vi "log analysis_gps.vi"() -> ()   [LabVIEW 2018] (continued)
robot status\t98.646724\t124.090697\t7.903900\t-0.225779\t-0.330995\t22.927991\t0.293000\t0.000000\n\t\n15:11:22.4\tlog_raw\tgps_raw\t#DUALANTENNAHEADINGA,USB3,0,48.5,FINESTEERING,2107,281500.400,02008000,d426,15824;SOL_COMPUTED,L1_FLOAT,-1.000000000,46.407375336,-16.426940918,0.0,360.000000000,180.000000000,\"631T\",18,7,7,7,04,00,20,02*243e6382\n\tsystem status\tnormal 2 28.200000 0 0\trobot status\t98.785641\t124.138688\t7.903500\t-0.300068\t-0.288771\t22.729309\t0.300000\t0.001000\n\t\n15:11:22.9\tlog_raw\tgps_raw\t#DUALANTENNAHEADINGA,USB3,0,48.5,FINESTEERING,2107,281500.900,02008000,d426,15824;SOL_COMPUTED,L1_FLOAT,-1.000000000,46.192268372,-15.498413086,0.0,360.000000000,180.000000000,\"631T\",17,7,7,7,04,00,20,02*d63e23bb\n\tsystem status\tnormal 2 28.200000 0 0\trobot status\t98.919497\t124.181484\t7.902700\t-0.165116\t-0.303857\t22.510660\t0.296000\t-0.008000\n\t\n15:11:23.4\tlog_raw\tgps_raw\t#DUALANTENNAHEADINGA,USB3,0,48.5,FINESTEERING,2107,281501.400,02008000,d426,15824;SOL_COMPUTED,L1_FLOAT,-1.000000000,48.142848969,-21.188415527,0.0,360.000000000,180.000000000,\"631T\",17,7,7,7,04,00,20,02*7f9c1701\n\tsystem status\tnormal 2 28.200000 0 0\trobot status\t99.058497\t124.228185\t7.902400\t-0.026703\t-0.321474\t22.196441\t0.302000\t-0.008000\n\t\n15:11:23.9\tlog_raw\tgps_raw\t#DUALANTENNAHEADINGA,USB3,0,48.5,FINESTEERING,2107,281501.900,02008000,d426,15824;SOL_COMPUTED,L1_FLOAT,-1.000000000,48.243919373,-21.323577881,0.0,360.000000000,180.000000000,\"631T\",18,7,7,7,04,00,20,02*9b797559\n\tsystem status\tnormal 2 28.200000 0 0\trobot status\t99.198528\t124.274008\t7.901400\t0.031138\t-0.500462\t21.899605\t0.292000\t-0.018000\n\t\n15:11:24.4\tlog_raw\tgps_raw\t#DUALANTENNAHEADINGA,USB3,0,51.0,FINESTEERING,2107,281502.400,02000000,d426,15824;SOL_COMPUTED,L1_FLOAT,-1.000000000,54.417652130,-31.199645996,0.0,360.000000000,180.000000000,\"631T\",17,7,7,7,04,00,20,02*139cf8a7\n\tsystem status\tnormal 2 28.200000 0 0\trobot status\t99.336569\t124.322202\t7.900100\t-0.095211\t-0.669796\t21.458028\t0.235000\t-0.092000\n\t\n15:11:24.9\tlog_raw\tgps_raw\t\tsystem status\tnormal 2 28.100000 0 0\trobot status\t99.472138\t124.367009\t7.899200\t-0.169834\t-0.458120\t20.912602\t0.280000\t-0.035000\n\t\n15:11:25.4\tlog_raw\tgps_raw\t\tsystem status\tnormal 2 28.200000 0 0\trobot status\t99.609993\t124.411117\t7.898200\t-0.103974\t-0.294964\t20.251587\t0.290000\t-0.052000\n\t\n15:11:25.9\tlog_raw\tgps_raw\t\tsystem status\tnormal 2 28.100000 0 0\trobot status\t99.748652\t124.451922\t7.895200\t-0.029652\t-0.262619\t19.517331\t0.383000\t0.101000\n\t\n15:11:26.4\tlog_raw\tgps_raw\t\tsystem status\tnormal 2 28.100000 0 0\trobot status\t99.889419\t124.493856\t7.892100\t0.011105\t-0.261460\t18.582918\t0.286000\t-0.034000\n\t\n15:11:26.9\tlog_raw\tgps_raw\t#DUALANTENNAHEADINGA,USB3,0,51.0,FINESTEERING,2107,281504.900,02000000,d426,15824;SOL_COMPUTED,NARROW_FLOAT,-1.000000000,45.458030701,-24.170471191,0.0,349.614562988,180.000000000,\"631T\",18,7,7,7,04,00,20,03*3763f111\n\tsystem status\tnormal 2 28.000000 0 0\trobot status\t100.028200\t124.531303\t7.889700\t0.052509\t-0.445143\t17.486224\t0.246000\t-0.119000\n\t\n15:11:27.4\tlog_raw\tgps_raw\t\tsystem status\tnormal 2 28.000000 0 0\trobot status\t100.174107\t124.568549\t7.889400\t0.061035\t-0.832335\t16.254658\t0.300000\t-0.053000\n\t\n15:11:27.9\tlog_raw\tgps_raw\t\tsystem status\tnormal 2 28.000000 0 0\trobot status\t100.318986\t124.599317\t7.888100\t0.214199\t-1.050680\t15.191319\t0.290000\t-0.056000\n\t\n15:11:28.4\tlog_raw\tgps_raw\t#DUALANTENNAHEADINGA,USB3,0,47.0,FINESTEERING,2107,281506.400,02000000,d426,15824;SOL_COMPUTED,L1_FLOAT,-1.000000000,47.490772247,-15.120605469,0.0,360.000000000,180.000000000,\"631T\",20,7,7,7,04,00,20,02*6c842724\n\tsystem status\tnormal 2 28.000000 0 0\trobot status\t100.462357\t124.629809\t7.887200\t0.132799\t-1.007596\t14.087784\t0.295000\t-0.054000\n\t\n15:11:28.9\tlog_raw\tgps_raw\t#DUALANTENNAHEADINGA,USB3,0,47.0,FINESTEERING,2107,281506.900,02000000,d426,15824;SOL_COMPUTED,L1_FLOAT,-1.000000000,47.711154938,-15.635345459,0.0,360.000000000,180.000000000,\"631T\",18,7,7,7,04,00,20,02*a44c5d4d\n\tsystem status\tnormal 2 28.000000 0 0\trobot status\t100.606200\t124.656880\t7.884400\t-0.072719\t-0.959328\t13.073074\t0.251000\t-0.099000\n\t\n15:11:29.4\tlog_raw\tgps_raw\t#DUALANTENNAHEADINGA,USB3,0,47.5,FINESTEERING,2107,281507.400,02000000,d426,15824;SOL_COMPUTED,NARROW_FLOAT,-1.000000000,42.099899292,-18.667358398,0.0,341.481109619,180.000000000,\"631T\",17,7,7,7,04,00,20,03*b5db1bef\n\tsystem status\tnormal 2 28.000000 0 0\trobot status\t100.748865\t124.681433\t7.880500\t5.282500E-5\t-0.839396\t12.187824\t0.258000\t-0.078000\n\t\n15:11:29.9\tlog_raw\tgps_raw\t#INSPVAXA,USB3,0,47.5,FINESTEERING,2107,281507.950,02000000,471d,15824;INS_ALIGNMENT_COMPLETE,INS_RTKFIXED,37.37125380804,126.72197426812,7.8769,22.3000,-0.0203,0.2606,-0.0150,0.201245645,-0.677592145,78.627863448,0.4158,0.2828,0.5148,0.1162,0.0939,0.0753,0.2087,0.2003,5.2095,0f000001,0*4e226b57\n\tsystem status\tnormal 2 28.000000 0 0\trobot status\t100.905195\t124.702970\t7.876900\t0.201246\t-0.677592\t11.372137\t0.348000\t0.066000\n\t\n15:11:30.4\tlog_raw\tgps_raw\t\tsystem status\tnormal 2 28.000000 0 0\trobot status\t101.036080\t124.720598\t7.875000\t0.298084\t-0.652481\t10.723363\t0.297000\t-0.011000\n\t\n15:11:30.9\tlog_raw\tgps_raw\t#DUALANTENNAHEADINGA,USB3,0,49.0,FINESTEERING,2107,281508.900,02000000,d426,15824;SOL_COMPUTED,L1_FLOAT,-1.000000000,44.870548248,-15.658569336,0.0,360.000000000,180.000000000,\"631T\",16,7,7,7,04,00,20,02*b0c8f4ea\n\tsystem status\tnormal 2 28.100000 0 0\trobot status\t101.181077\t124.738550\t7.872400\t0.183203\t-0.630905\t10.014511\t0.311000\t0.003000\n\t\n15:11:31.4\tlog_raw\tgps_raw\t#DUALANTENNAHEADINGA,USB3,0,48.0,FINESTEERING,2107,281509.400,02000000,d426,15824;SOL_COMPUTED,NARROW_FLOAT,-1.000000000,43.414321899,-11.001037598,0.0,331.000732422,180.000000000,\"631T\",16,7,7,7,04,00,20,03*47deaf74\n\tsystem status\tnormal 2 28.100000 0 0\trobot status\t101.323239\t124.757427\t7.870200\t0.032270\t-0.532308\t9.546934\t0.287000\t-0.036000\n\t\n15:11:31.9\tlog_raw\tgps_raw\t#INSPVAXA,USB3,0,48.0,FINESTEERING,2107,281509.950,02000000,471d,15824;INS_ALIGNMENT_COMPLETE,INS_RTKFIXED,37.37125445097,126.72198074425,7.8673,22.3000,-0.0085,0.2660,-0.0026,-0.121772207,-0.607137029,81.065804036,0.4154,0.2822,0.5141,0.1167,0.0945,0.0753,0.2051,0.1982,5.2122,0f000001,0*3f1eba48\n\tsystem status\tnormal 2 28.100000 0 0\trobot status\t101.478840\t124.774319\t7.867300\t-0.121772\t-0.607137\t8.934196\t0.256000\t-0.074000\n\t\n15:11:32.4\tlog_raw\tgps_raw\t\tsystem status\tnormal 2 28.200000 0 0\trobot status\t101.608572\t124.787896\t7.865000\t0.007019\t-0.726552\t8.514396\t0.304000\t-0.013000\n\t\n15:11:32.9\tlog_raw\tgps_raw\t#INSPVAXA,USB3,0,49.0,FINESTEERING,2107,281510.950,02000000,471d,15824;INS_ALIGNMENT_COMPLETE,INS_RTKFIXED,37.37125469386,126.72198394017,7.8637,22.3000,-0.0196,0.2391,0.0072,0.076200497,-0.660108168,81.872681824,0.4156,0.2817,0.5136,0.1168,0.0948,0.0753,0.2032,0.1971,5.2137,0f000001,0*0481949b\n\tsystem status\tnormal 2 28.200000 0 0\trobot status\t101.761929\t124.801272\t7.863700\t0.076200\t-0.660108\t8.127318\t0.235000\t-0.092000\n\t\n15:11:33.4\tlog_raw\tgps_raw\t#DUALANTENNAHEADINGA,USB3,0,46.5,FINESTEERING,2107,281511.400,02000000,d426,15824;SOL_COMPUTED,L1_FLOAT,-1.000000000,48.665706635,-11.851898193,0.0,360.000000000,180.000000000,\"631T\",23,7,7,7,04,00,20,02*002e390f\n\tsystem status\tnormal 2 28.200000 0 0\trobot status\t101.889941\t124.812552\t7.861000\t0.084258\t-0.827369\t7.753561\t0.346000\t0.053000\n\t\n15:11:33.9\tlog_raw\tgps_raw\t#DUALANTENNAHEADINGA,USB3,0,46.5,FINESTEERING,2107,281511.900,02000000,d426,15824;SOL_COMPUTED,L1_FLOAT,-1.000000000,49.675540924,-13.921539307,0.0,360.000000000,180.000000000,\"631T\",22,7,7,7,04,00,20,02*d8f1bbd6\n\tsystem status\tnormal 2 28.200000 0 0\trobot status\t102.034901\t124.823355\t7.857600\t0.091248\t-1.206859\t7.443421\t0.347000\t0.065000\n\t\n15:11:34.4\tlog_raw\tgps_raw\t\tsystem status\tnormal 2 28.200000 0 0\trobot status\t102.180454\t124.835621\t7.854200\t0.123162\t-1.430289\t7.169938\t0.298000\t-0.010000\n\t\n15:11:34.9\tlog_raw\tgps_raw\t\tsystem status\tnormal 2 28.200000 0 0\trobot status\t102.318034\t124.846412\t7.851300\t0.027853\t-1.487298\t6.927742\t0.312000\t-0.001000\n\t\n15:11:35.4\tlog_raw\tgps_raw\t\tsystem status\tnormal 2 28.200000 0 0\trobot status\t102.466690\t124.857181\t7.847700\t0.249609\t-1.679451\t6.774904\t0.306000\t-0.003000\n\t\n15:11:35.9\tlog_raw\tgps_raw\t#DUALANTENNAHEADINGA,USB3,0,49.5,FINESTEERING,2107,281513.900,02000000,d426,15824;SOL_COMPUTED,NARROW_FLOAT,-1.000000000,44.284626007,-19.218811035,0.0,360.000000000,180.000000000,\"631T\",20,7,7,7,04,00,20,02*521f05df\n\tsystem status\tnormal 2 28.200000 0 0\trobot status\t102.608975\t124.865714\t7.841900\t0.369371\t-1.895271\t6.487621\t0.281000\t-0.030000\n\t\n15:11:36.4\tlog_raw\tgps_raw\t#INSPVAXA,USB3,0,49.5,FINESTEERING,2107,281514.450,02000000,471d,15824;INS_ALIGNMENT_COMPLETE,INS_RTKFIXED,37.37125536287,126.72199528915,7.8355,22.3000,-0.0378,0.2111,0.0002,0.439353966,-1.869293948,83.706823159,0.4159,0.2810,0.5124,0.1164,0.0945,0.0753,0.1954,0.1923,5.2170,0f000001,0*665bd911\n\tsystem status\tnormal 2 28.200000 0 0\trobot status\t102.767204\t124.875510\t7.835500\t0.439354\t-1.869294\t6.293177\t0.346000\t0.076000\n\t\n15:11:36.9\tlog_raw\tgps_raw\t\tsystem status\tnormal 2 28.200000 0 0\trobot status\t102.889412\t124.880327\t7.832000\t0.623351\t-1.525820\t6.078909\t0.311000\t-0.001000\n\t\n15:11:37.4\tlog_raw\tgps_raw\t#DUALANTENNAHEADINGA,USB3,0,49.0,FINESTEERING,2107,281515.400,02000000,d426,15824;SOL_COMPUTED,L1_FLOAT,-1.000000000,38.143417358,-18.359069824,0.0,274.915802002,180.000000000,\"631T\",19,9,9,9,04,00,20,22*781bfffa\n\tsystem status\tnormal 2 28.200000 0 0\trobot status\t103.038346\t124.886833\t7.827900\t0.687382\t-1.870260\t5.833892\t0.299000\t-0.009000\n\t\n15:11:37.9\tlog_raw\tgps_raw\t#INSPVAXA,USB3,0,49.0,FINESTEERING,2107,281515.950,02000000,471d,15824;INS_ALIGNMENT_COMPLETE,INS_RTKFIXED,37.37125550223,126.72200026219,7.8204,22.3000,-0.0297,0.2447,-0.0075,0.993050035,-2.146972664,84.455014366,0.4154,0.2808,0.5121,0.1158,0.0940,0.0753,0.1936,0.1911,5.2166,0f000001,0*f4a4a55a\n\tsystem status\tnormal 2 28.200000 0 0\trobot status\t103.207707\t124.890971\t7.820400\t0.993050\t-2.146973\t5.544986\t0.330000\t0.040000\n\t\n15:11:38.4\tlog_raw\tgps_raw\t\tsystem status\tnormal 2 28.200000 0 0\trobot status\t103.325362\t124.896784\t7.815000\t0.884537\t-1.973530\t5.489952\t0.303000\t-0.002000\n\t\n15:11:38.9\tlog_raw\tgps_raw\t#INSPVAXA,USB3,0,49.5,FINESTEERING,2107,281516.950,02000000,471d,15824;INS_ALIGNMENT_COMPLETE,INS_RTKFIXED,37.37125561676,126.72200346260,7.8093,22.3000,-0.0298,0.2388,-0.0036,0.877000312,-2.356206716,84.738207188,0.4150,0.2807,0.5119,0.1151,0.0935,0.0753,0.1918,0.1900,5.2169,0f000001,0*302168dd\n\tsystem status\tnormal 2 28.200000 0 0\trobot status\t103.491194\t124.903679\t7.809300\t0.877000\t-2.356207\t5.261793\t0.283000\t-0.020000\n\t\n15:11:39.4\tlog_raw\tgps_raw\t\tsystem status\tnormal 2 28.200000 0 0\trobot status\t103.620894\t124.907401\t7.804000\t1.139173\t-2.452817\t5.195560\t0.315000\t0.002000\n\t\n15:11:39.9\tlog_raw\tgps_raw\t#INSPVAXA,USB3,0,49.0,FINESTEERING,2107,281517.950,02000000,471d,15824;INS_ALIGNMENT_COMPLETE,INS_RTKFIXED,37.37125568444,126.72200682151,7.7945,22.3000,-0.0192,0.2217,-0.0192,1.425946451,-2.539207007,85.090836671,0.4150,0.2807,0.5120,0.1146,0.0931,0.0754,0.1902,0.1890,5.2177,0f000001,0*9a7264e1\n\tsystem status\tnormal 2 28.200000 0 0\trobot status\t103.788721\t124.911187\t7.794500\t1.425946\t-2.539207\t4.909163\t0.292000\t-0.003000\n\t\n15:11:40.4\tlog_raw\tgps_raw\t#DUALANTENNAHEADINGA,USB3,0,47.0,FINESTEERING,2107,281518.400,02000000,d426,15824;SOL_COMPUTED,L1_FLOAT,-1.000000000,42.740367889,-32.075164795,0.0,319.860687256,180.000000000,\"631T\",19,9,9,9,04,00,20,22*d53a90ac\n\tsystem status\tnormal 2 28.200000 0 0\trobot status\t103.913646\t124.913656\t7.788400\t1.548086\t-2.511237\t4.765725\t0.294000\t-0.015000\n\t\n15:11:40.9\tlog_raw\tgps_raw\t#INSPVAXA,USB3,0,47.0,FINESTEERING,2107,281518.950,02000000,471d,15824;INS_ALIGNMENT_COMPLETE,INS_RTKFIXED,37.37125573981,126.72201005340,7.7819,22.3000,-0.0255,0.2627,-0.0105,1.331964681,-2.358060852,85.490717042,0.4145,0.2807,0.5123,0.1139,0.0926,0.0754,0.1888,0.1882,5.2187,0f000001,0*a7b8d42f\n\tsystem status\tnormal 2 28.200000 0 0\trobot status\t104.074997\t124.917328\t7.781900\t1.331965\t-2.358061\t4.509283\t0.295000\t-0.010000\n\t\n15:11:41.4\tlog_raw\tgps_raw\t\tsystem status\tnormal 2 28.200000 0 0\trobot status\t104.206873\t124.921189\t7.776100\t1.272173\t-2.469468\t4.361029\t0.303000\t-0.005000\n\t\n15:11:41.9\tlog_raw\tgps_raw\t#DUALANTENNAHEADINGA,USB3,0,48.5,FINESTEERING,2107,281519.900,02000000,d426,15824;SOL_COMPUTED,L1_FLOAT,-1.000000000,50.327861786,-37.477569580,0.0,318.157135010,180.000000000,\"631T\",19,6,6,6,04,00,20,02*633b419f\n\tsystem status\tnormal 2 28.200000 0 0\trobot status\t104.351513\t124.926330\t7.769800\t0.918221\t-2.120112\t4.233972\t0.281000\t-0.028000\n\t\n15:11:42.4\tlog_raw\tgps_raw\t#INSPVAXA,USB3,0,50.5,FINESTEERING,2107,281520.450,02000000,471d,15824;INS_ALIGNMENT_COMPLETE,INS_RTKFIXED,37.37125585823,126.72201493380,7.7618,22.3000,-0.0241,0.3156,-0.0229,0.726950226,-1.736335122,85.946194280,0.4135,0.2799,0.5121,0.1130,0.0919,0.0756,0.1864,0.1868,5.2210,0f000001,0*82c9f176\n\tsystem status\tnormal 2 28.200000 0 0\trobot status\t104.507294\t124.930466\t7.761800\t0.726950\t-1.736335\t4.053806\t0.309000\t-0.011000\n\t\n15:11:42.9\tlog_raw\tgps_raw\t#INSPVAXA,USB3,0,50.5,FINESTEERING,2107,281520.950,02000000,471d,15824;INS_ALIGNMENT_COMPLETE,INS_RTKFIXED,37.37125587974,126.72201671987,7.7507,22.3000,-0.0399,0.2427,-0.0046,0.656221205,-1.866737279,86.202077970,0.4135,0.2799,0.5121,0.1130,0.0919,0.0756,0.1864,0.1868,5.2210,0f000001,0*df1ef1f5\n\tsystem status\tnormal 2 28.200000 0 0\trobot status\t104.665502\t124.932851\t7.750700\t0.656221\t-1.866737\t3.797922\t0.277000\t-0.018000\n\t\n15:11:43.4\tlog_raw\tgps_raw\t\tsystem status\tnormal 2 28.200000 0 0\trobot status\t104.773354\t124.932494\t7.745800\t0.650732\t-1.574531\t3.665864\t0.288000\t0.009000\n\t\n15:11:43.9\tlog_raw\tgps_raw\t#INSPVAXA,USB3,0,46.5,FINESTEERING,2107,281521.950,02000000,471d,15824;INS_ALIGNMENT_COMPLETE,INS_RTKFIXED,37.37125587376,126.72201976127,7.7406,22.3000,-0.0074,0.2755,0.0027,0.545815584,-0.620038116,86.574318389,0.4139,0.2794,0.5123,0.1122,0.0918,0.0756,0.1854,0.1863,5.2222,0f000001,0*d388b8b0\n\tsystem status\tnormal 2 28.200000 0 0\trobot status\t104.934904\t124.932184\t7.740600\t0.545816\t-0.620038\t3.425682\t0.297000\t-0.002000\n\t\n15:11:44.4\tlog_raw\tgps_raw\t#INSPVAXA,USB3,0,50.0,FINESTEERING,2107,281522.450,02000000,471d,15824;INS_ALIGNMENT_COMPLETE,INS_RTKFIXED,37.37125594460,126.72202128419,7.7372,22.3000,-0.0117,0.2731,-0.0129,-0.654259534,-0.666330623,86.875849096,0.4136,0.2787,0.5123,0.1124,0.0922,0.0756,0.1845,0.1859,5.2224,0f000001,0*d87bbb5d\n\tsystem status\tnormal 2 28.200000 0 0\trobot status\t105.069802\t124.940044\t7.737200\t-0.654260\t-0.666331\t3.124151\t0.300000\t0.002000\n\t\n15:11:44.9\tlog_raw\tgps_raw\t#INSPVAXA,USB3,0,50.0,FINESTEERING,2107,281522.950,02000000,471d,15824;INS_ALIGNMENT_COMPLETE,INS_RTKFIXED,37.37125596414,126.72202295836,7.7342,22.3000,-0.0333,0.2828,-0.0046,-1.065587948,-0.382081597,87.029767697,0.4136,0.2787,0.5123,0.1124,0.0922,0.0756,0.1845,0.1859,5.2224,0f000001,0*2edab05f\n\tsystem status\tnormal 2 28.200000 0 0\trobot status\t105.218097\t124.942211\t7.734200\t-1.065588\t-0.382082\t2.970232\t0.302000\t-0.002000\n\t\n15:11:45.4\tlog_raw\tgps_raw\t#INSPVAXA,USB3,0,50.0,FINESTEERING,2107,281523.450,02000000,471d,15824;INS_ALIGNMENT_COMPLETE,INS_RTKFIXED,37.37125596415,126.72202454079,7.7319,22.3000,-0.0484,0.2411,-0.0123,-1.089747503,0.421440588,87.147048457,0.4141,0.2781,0.5123,0.1124,0.0923,0.0755,0.1837,0.1856,5.2192,0f000001,0*53e95b2b\n\tsystem status\tnormal 2 28.200000 0 0\trobot status\t105.358266\t124.942210\t7.731900\t-1.089748\t0.421441\t2.852952\t0.294000\t0.001000\n\t\n15:11:45.9\tlog_raw\tgps_raw\t#INSPVAXA,USB3,0,50.0,FINESTEERING,2107,281523.950,02000000,471d,15824;INS_ALIGNMENT_COMPLETE,INS_RTKFIXED,37.37125592914,126.72202612283,7.7345,22.3000,-0.0454,0.2984,-0.0075,-0.788968159,0.571056615,87.325442989,0.4141,0.2781,0.5123,0.1124,0.0923,0.0755,0.1837,0.1856,5.2192,0f000001,0*39ccc3b7\n\tsystem status\tnormal 2 28.200000 0 0\trobot status\t105.498400\t124.938323\t7.734500\t-0.788968\t0.571057\t2.674557\t0.312000\t-0.009000\n\t\n15:11:46.4\tlog_raw\tgps_raw\t#INSPVAXA,USB3,0,50.0,FINESTEERING,2107,281524.450,02000000,471d,15824;INS_ALIGNMENT_COMPLETE,INS_RTKFIXED,37.37125593181,126.72202769254,7.7370,22.3000,-0.0382,0.2867,-0.0035,-1.197739356,0.920892759,87.655051313,0.4147,0.2775,0.5122,0.1123,0.0915,0.0754,0.1830,0.1854,5.2111,0f000001,0*f9d72c69\n\tsystem status\tnormal 2 28.200000 0 0\trobot status\t105.637443\t124.938618\t7.737000\t-1.197739\t0.920893\t2.344949\t0.309000\t-0.005000\n\t\n15:11:46.9\tlog_raw\tgps_raw\t#INSPVAXA,USB3,0,50.0,FINESTEERING,2107,281524.950,02000000,471d,15824;INS_ALIGNMENT_COMPLETE,INS_RTKFIXED,37.37125591109,126.72202930356,7.7399,22.3000,-0.0391,0.2791,0.0008,-1.548464832,1.177525409,87.896240869,0.4147,0.2775,0.5122,0.1123,0.0915,0.0754,0.1830,0.1854,5.2111,0f000001,0*83d571d9\n\tsystem status\tnormal 2 28.200000 0 0\trobot status\t105.780144\t124.936316\t7.739900\t-1.548465\t1.177525\t2.103759\t0.307000\t-0.003000\n\t\n15:11:47.4\tlog_raw\tgps_raw\t\tsystem status\tnormal 2 28.200000 0 0\trobot status\t105.910401\t124.935971\t7.743500\t-1.684978\t1.371222\t1.943675\t0.296000\t0.003000\n\t\n15:11:47.9\tlog_raw\tgps_raw\t\tsystem status\tnormal 2 28.200000 0 0\trobot status\t106.056063\t124.933146\t7.747400\t-1.614315\t1.306008\t1.765428\t0.294000\t0.000000\n\t\n15:11:48.4\tlog_raw\tgps_raw\t#INSPVAXA,USB3,0,48.5,FINESTEERING,2107,281526.450,02000000,471d,15824;INS_ALIGNMENT_COMPLETE,INS_RTKFIXED,37.37125584524,126.72203425117,7.7504,22.3000,-0.0601,0.2713,0.0036,-1.381885120,0.929156206,88.315257538,0.4157,0.2770,0.5121,0.1113,0.0909,0.0752,0.1819,0.1851,5.1872,0f000001,0*291f5036\n\tsystem status\tnormal 2 28.200000 0 0\trobot status\t106.218395\t124.929002\t7.750400\t-1.381885\t0.929156\t1.684742\t0.293000\t-0.004000\n\t\n15:11:48.9\tlog_raw\tgps_raw\t#INSPVAXA,USB3,0,48.5,FINESTEERING,2107,281526.950,02000000,471d,15824;INS_ALIGNMENT_COMPLETE,INS_RTKFIXED,37.37125579589,126.72203592362,7.7537,22.3000,-0.0480,0.2913,0.0058,-1.173614643,0.491373435,88.468098550,0.4157,0.2770,0.5121,0.1113,0.0909,0.0752,0.1819,0.1851,5.1872,0f000001,0*d2925fbc\n\tsystem status\tnormal 2 28.200000 0 0\trobot status\t106.366538\t124.923523\t7.753700\t-1.173615\t0.491373\t1.531901\t0.306000\t0.008000\n\t\n15:11:49.4\tlog_raw\tgps_raw\t\tsystem status\tnormal 2 28.200000 0 0\trobot status\t106.498057\t124.921350\t7.758600\t-1.119985\t0.342214\t1.463884\t0.297000\t0.006000\n\t\n15:11:49.9\tlog_raw\tgps_raw\t#INSPVAXA,USB3,0,48.0,FINESTEERING,2107,281527.950,02000000,471d,15824;INS_ALIGNMENT_COMPLETE,INS_RTKFIXED,37.37125572987,126.72203920387,7.7658,22.3000,-0.0524,0.2827,0.0097,-1.037615200,0.271270878,88.658127603,0.4153,0.2771,0.5121,0.1104,0.0905,0.0752,0.1816,0.1850,5.1752,0f000001,0*cc65e324\n\tsystem status\tnormal 2 28.200000 0 0\trobot status\t106.657097\t124.916193\t7.765800\t-1.037615\t0.271271\t1.341872\t0.302000\t0.006000\n\t\n15:11:50.4\tlog_raw\tgps_raw\t#INSPVAXA,USB3,0,50.0,FINESTEERING,2107,281528.450,02000000,471d,15824;INS_ALIGNMENT_COMPLETE,INS_RTKFIXED,37.37125569644,126.72204084208,7.7707,22.3000,-0.0559,0.2951,0.0043,-0.934405455,0.587306829,88.715451510,0.4138,0.2768,0.5118,0.1101,0.0902,0.0751,0.1812,0.1850,5.1681,0f000001,0*38aa8fdd\n\tsystem status\tnormal 2 28.200000 0 0\trobot status\t106.802207\t124.912480\t7.770700\t-0.934405\t0.587307\t1.284548\t0.301000\t0.002000\n\t\n15:11:50.9\tlog_raw\tgps_raw\t#INSPVAXA,USB3,0,50.0,FINESTEERING,2107,281528.950,02000000,471d,15824;INS_ALIGNMENT_COMPLETE,INS_RTKFIXED,37.37125565087,126.72204247728,7.7739,22.3000,-0.0479,0.2916,0.0001,-0.888338031,0.781445457,88.804413207,0.4138,0.2768,0.5118,0.1101,0.0902,0.0751,0.1812,0.1850,5.1681,0f000001,0*a995e794\n\tsystem status\tnormal 2 28.200000 0 0\trobot status\t106.947051\t124.907421\t7.773900\t-0.888338\t0.781445\t1.195587\t0.298000\t0.004000\n\t\n15:11:51.4\tlog_raw\tgps_raw\t#INSPVAXA,USB3,0,45.5,FINESTEERING,2107,281529.450,02000000,471d,15824;INS_ALIGNMENT_COMPLETE,INS_RTKFIXED,37.37125561815,126.72204405961,7.7805,22.3000,-0.0427,0.2707,0.0059,-0.985512427,0.998310951,88.869085357,0.4125,0.2769,0.5116,0.1099,0.0902,0.0751,0.1810,0.1850,5.1659,0f000001,0*0269fb35\n\tsystem status\tnormal 2 28.200000 0 0\trobot status\t107.087211\t124.903788\t7.780500\t-0.985512\t0.998311\t1.130915\t0.294000\t-0.009000\n\t\n15:11:51.9\tlog_raw\tgps_raw\t#INSPVAXA,USB3,0,45.5,FINESTEERING,2107,281529.950,02000000,471d,15824;INS_ALIGNMENT_COMPLETE,INS_RTKFIXED,37.37125556208,126.72204568853,7.7886,22.3000,-0.0448,0.2875,0.0039,-0.937316119,0.971606302,88.876668498,0.4125,0.2769,0.5116,0.1099,0.0902,0.0751,0.1810,0.1850,5.1659,0f000001,0*914c1aec\n\tsystem status\tnormal 2 28.200000 0 0\trobot status\t107.231498\t124.897563\t7.788600\t-0.937316\t0.971606\t1.123332\t0.298000\t-0.003000\n\t\n15:11:52.4\tlog_raw\tgps_raw\t#INSPVAXA,USB3,0,49.0,FINESTEERING,2107,281530.450,02000000,471d,15824;INS_ALIGNMENT_COMPLETE,INS_RTKFIXED,37.37125551286,126.72204733678,7.7958,22.3000,-0.0391,0.2940,0.0024,-0.847859787,0.758698314,88.842002918,0.4116,0.2768,0.5112,0.1098,0.0901,0.0751,0.1808,0.1849,5.1659,0f000001,0*a7731e83\n\tsystem status\tnormal 2 28.200000 0 0\trobot status\t107.377497\t124.892099\t7.795800\t-0.847860\t0.758698\t1.157997\t0.300000\t0.001000\n\t\n15:11:52.9\tlog_raw\tgps_raw\t#INSPVAXA,USB3,0,49.0,FINESTEERING,2107,281530.950,02000000,471d,15824;INS_ALIGNMENT_COMPLETE,INS_RTKFIXED,37.37125545025,126.72204900061,7.8022,22.3000,-0.0360,0.2787,-0.0016,-0.812645512,0.794768831,88.914177046,0.4116,0.2768,0.5112,0.1098,0.0901,0.0751,0.1808,0.1849,5.1659,0f000001,0*55377a3b\n\tsystem status\tnormal 2 28.200000 0 0\trobot status\t107.524877\t124.885148\t7.802200\t-0.812646\t0.794769\t1.085823\t0.296000\t0.003000\n\t\n15:11:53.4\tlog_raw\tgps_raw\t#INSPVAXA,USB3,0,48.5,FINESTEERING,2107,281531.450,02000000,471d,15824;INS_ALIGNMENT_COMPLETE,INS_RTKFIXED,37.37125540137,126.72205063289,7.8075,22.3000,-0.0425,0.2797,0.0032,-0.889554517,0.869596367,88.992176965,0.4129,0.2847,0.5220,0.1101,0.0915,0.0760,0.1808,0.1849,5.1672,0f000001,0*7c4913e5\n\tsystem status\tnormal 2 28.200000 0 0\trobot status\t107.669461\t124.879721\t7.807500\t-0.889555\t0.869596\t1.007823\t0.302000\t0.002000\n\t\n15:11:53.9\tlog_raw\tgps_raw\t#INSPVAXA,USB3,0,48.5,FINESTEERING,2107,281531.950,02000000,471d,15824;INS_ALIGNMENT_COMPLETE,INS_RTKFIXED,37.37125534314,126.72205229379,7.8137,22.3000,-0.0465,0.3065,0.0071,-1.008380878,0.751327706,89.074001876,0.4129,0.2847,0.5220,0.1101,0.0915,0.0760,0.1808,0.1849,5.1672,0f000001,0*42202879\n\tsystem status\tnormal 2 28.200000 0 0\trobot status\t107.816581\t124.873257\t7.813700\t-1.008381\t0.751328\t0.925998\t0.302000\t0.002000\n\t\n15:11:54.4\tlog_raw\tgps_raw\t#INSPVAXA,USB3,0,47.5,FINESTEERING,2107,281532.450,02000000,471d,15824;INS_ALIGNMENT_COMPLETE,INS_RTKFIXED,37.37125529086,126.72205393210,7.8208,22.3000,-0.0380,0.2964,0.0024,-1.066354382,0.654899534,89.120116128,0.4138,0.2906,0.5321,0.1104,0.0921,0.0766,0.1807,0.1849,5.1689,0f000001,0*be946886\n\tsystem status\tnormal 2 28.200000 0 0\trobot status\t107.961700\t124.867452\t7.820800\t-1.066354\t0.654900\t0.879884\t0.299000\t0.003000\n\t\n15:11:54.9\tlog_raw\tgps_raw\t#INSPVAXA,USB3,0,47.5,FINESTEERING,2107,281532.950,02000000,471d,15824;INS_ALIGNMENT_COMPLETE,INS_RTKFIXED,37.37125523061,126.72205555403,7.8287,22.3000,-0.0378,0.2817,0.0049,-1.169453281,0.642583735,89.146408526,0.4138,0.2906,0.5321,0.1104,0.0921,0.0766,0.1807,0.1849,5.1689,0f000001,0*6f8607ae\n\tsystem status\tnormal 2 28.200000 0 0\trobot status\t108.105368\t124.860764\t7.828700\t-1.169453\t0.642584\t0.853591\t0.295000\t0.002000\n\t\n15:11:55.4\tlog_raw\tgps_raw\t#INSPVAXA,USB3,0,48.5,FINESTEERING,2107,281533.450,02000000,471d,15824;INS_ALIGNMENT_COMPLETE,INS_RTKFIXED,37.37125517665,126.72205724840,7.8341,22.3000,-0.0370,0.2921,0.0139,-1.096637131,0.532202635,89.160335545,0.4113,0.2846,0.5267,0.1101,0.0906,0.0761,0.1804,0.1849,5.1704,0f000001,0*30c8b167\n\tsystem status\tnormal 2 28.200000 0 0\trobot status\t108.255452\t124.854773\t7.834100\t-1.096637\t0.532203\t0.839664\t0.304000\t0.000000\n\t\n15:11:55.9\tlog_raw\tgps_raw\t#INSPVAXA,USB3,0,48.5,FINESTEERING,2107,281533.950,02000000,471d,15824;INS_ALIGNMENT_COMPLETE,INS_RTKFIXED,37.37125511841,126.72205890911,7.8393,22.3000,-0.0280,0.2944,0.0195,-1.130148525,0.576717755,89.139209909,0.4113,0.2846,0.5267,0.1101,0.0906,0.0761,0.1804,0.1849,5.1704,0f000001,0*9cf16a0c\n\tsystem status\tnormal 2 28.200000 0 0\trobot status\t108.402555\t124.848307\t7.839300\t-1.130149\t0.576718\t0.860790\t0.304000\t-0.003000\n\t\n15:11:56.4\tlog_raw\tgps_raw\t#INSPVAXA,USB3,0,49.0,FINESTEERING,2107,281534.450,02000000,471d,15824;INS_ALIGNMENT_COMPLETE,INS_RTKFIXED,37.37125507853,126.72206052520,7.8451,22.3000,-0.0278,0.2839,0.0233,-1.120245446,0.696634414,89.152346595,0.4098,0.2808,0.5226,0.1101,0.0900,0.0757,0.1802,0.1849,5.1715,0f000001,0*4ae7b9de\n\tsystem status\tnormal 2 28.200000 0 0\trobot status\t108.545706\t124.843880\t7.845100\t-1.120245\t0.696634\t0.847653\t0.278000\t0.038000\n\t\n15:11:56.9\tlog_raw\tgps_raw\t\tsystem status\tnormal 2 28.200000 0 0\trobot status\t108.675907\t124.839047\t7.850800\t-1.049400\t0.685732\t0.841710\t0.256000\t0.060000\n\t\n15:11:57.4\tlog_raw\tgps_raw\t#INSPVAXA,USB3,0,48.5,FINESTEERING,2107,281535.450,02000000,471d,15824;INS_ALIGNMENT_COMPLETE,INS_RTKFIXED,37.37125500223,126.72206378998,7.8595,22.3000,-0.0263,0.2848,0.0309,-1.021616386,0.668311678,89.031237589,0.4086,0.2786,0.5193,0.1098,0.0898,0.0755,0.1801,0.1849,5.1718,0f000001,0*96cd35cb\n\tsystem status\tnormal 2 28.200000 0 0\trobot status\t108.834895\t124.835408\t7.859500\t-1.021616\t0.668312\t0.968762\t0.295000\t0.014000\n\t\n15:11:57.9\tlog_raw\tgps_raw\t#INSPVAXA,USB3,0,48.5,FINESTEERING,2107,281535.950,02000000,471d,15824;INS_ALIGNMENT_COMPLETE,INS_RTKFIXED,37.37125496736,126.72206538562,7.8673,22.3000,-0.0208,0.2826,0.0283,-0.984984816,0.649258027,88.926389870,0.4086,0.2786,0.5193,0.1098,0.0898,0.0755,0.1801,0.1849,5.1718,0f000001,0*d651761b\n\tsystem status\tnormal 2 28.200000 0 0\trobot status\t108.976234\t124.831536\t7.867300\t-0.984985\t0.649258\t1.073610\t0.295000\t0.021000\n\t\n15:11:58.4\tlog_raw\tgps_raw\t#INSPVAXA,USB3,0,43.0,FINESTEERING,2107,281536.450,02000000,471d,15824;INS_ALIGNMENT_COMPLETE,INS_RTKFIXED,37.37125494902,126.72206698066,7.8731,22.3000,-0.0263,0.2809,0.0211,-1.040366850,0.673880913,88.812825832,0.4080,0.2774,0.5168,0.1098,0.0898,0.0754,0.1801,0.1849,5.1719,0f000001,0*bc17f841\n\tsystem status\tnormal 2 28.200000 0 0\trobot status\t109.117520\t124.829498\t7.873100\t-1.040367\t0.673881\t1.187174\t0.354000\t-0.072000\n\t\n15:11:58.9\tlog_raw\tgps_raw\t#INSPVAXA,USB3,0,43.0,FINESTEERING,2107,281536.950,02000000,471d,15824;INS_ALIGNMENT_COMPLETE,INS_RTKFIXED,37.37125492336,126.72206864315,7.8782,22.3000,-0.0243,0.2721,0.0164,-1.054954219,0.518295221,88.745495992,0.4080,0.2774,0.5168,0.1098,0.0898,0.0754,0.1801,0.1849,5.1719,0f000001,0*93a4c9d5\n\tsystem status\tnormal 2 28.200000 0 0\trobot status\t109.264781\t124.826649\t7.878200\t-1.054954\t0.518295\t1.254504\t0.285000\t0.018000\n\t\n15:11:59.4\tlog_raw\tgps_raw\t#INSPVAXA,USB3,0,49.5,FINESTEERING,2107,281537.450,02000000,471d,15824;INS_ALIGNMENT_COMPLETE,INS_RTKFIXED,37.37125492115,126.72207026375,7.8826,22.3000,-0.0312,0.2819,0.0093,-1.140326521,0.505680826,88.594443704,0.4075,0.2769,0.5150,0.1098,0.0900,0.0754,0.1800,0.1848,5.1716,0f000001,0*0036ae1b\n\tsystem status\tnormal 2 28.200000 0 0\trobot status\t109.408331\t124.826402\t7.882600\t-1.140327\t0.505681\t1.405556\t0.293000\t0.027000\n\t\n15:11:59.9\tlog_raw\tgps_raw\t#INSPVAXA,USB3,0,49.5,FINESTEERING,2107,281537.950,02000000,471d,15824;INS_ALIGNMENT_COMPLETE,INS_RTKFIXED,37.37125491697,126.72207184054,7.8872,22.3000,-0.0272,0.2819,0.0040,-1.130976236,0.507935776,88.476377303,0.4075,0.2769,0.5150,0.1098,0.0900,0.0754,0.1800,0.1848,5.1716,0f000001,0*f6fa546b\n\tsystem status\tnormal 2 28.200000 0 0\trobot status\t109.548000\t124.825936\t7.887200\t-1.130976\t0.507936\t1.523623\t0.253000\t0.074000\n\t\n15:12:00.4\tlog_raw\tgps_raw\t#INSPVAXA,USB3,0,49.5,FINESTEERING,2107,281538.450,02000000,471d,15824;INS_ALIGNMENT_COMPLETE,INS_RTKFIXED,37.37125491162,126.72207343326,7.8918,22.3000,-0.0245,0.2815,0.0124,-1.153453506,0.493104111,88.435314047,0.4072,0.2765,0.5135,0.1099,0.0900,0.0754,0.1800,0.1848,5.1710,0f000001,0*5ae8f9c6\n\tsystem status\tnormal 2 28.200000 0 0\trobot status\t109.689081\t124.825340\t7.891800\t-1.153454\t0.493104\t1.564686\t0.252000\t0.064000\n\t\n15:12:00.9\tlog_raw\tgps_raw\t#INSPVAXA,USB3,0,49.5,FINESTEERING,2107,281538.950,02000000,471d,15824;INS_ALIGNMENT_COMPLETE,INS_RTKFIXED,37.37125490028,126.72207504818,7.8968,22.3000,-0.0236,0.2833,0.0059,-1.091251980,0.482969465,88.379863366,0.4072,0.2765,0.5135,0.1099,0.0900,0.0754,0.1800,0.1848,5.1710,0f000001,0*2ba689f0\n\tsystem status\tnormal 2 28.200000 0 0\trobot status\t109.832128\t124.824080\t7.896800\t-1.091252\t0.482969\t1.620137\t0.285000\t0.017000\n\t\n15:12:01.4\tlog_raw\tgps_raw\t#INSPVAXA,USB3,0,48.5,FINESTEERING,2107,281539.450,02000000,471d,15824;INS_ALIGNMENT_COMPLETE,INS_RTKFIXED,37.37125490824,126.72207664117,7.9004,22.3000,-0.0216,0.2784,0.0079,-1.109314476,0.482411091,88.340192961,0.4069,0.2763,0.5124,0.1098,0.0900,0.0754,0.1799,0.1848,5.1698,0f000001,0*8761aced\n\tsystem status\tnormal 2 28.200000 0 0\trobot status\t109.973232\t124.824961\t7.900400\t-1.109314\t0.482411\t1.659807\t0.284000\t0.023000\n\t\n15:12:01.9\tlog_raw\tgps_raw\t#INSPVAXA,USB3,0,48.5,FINESTEERING,2107,281539.950,02000000,471d,15824;INS_ALIGNMENT_COMPLETE,INS_RTKFIXED,37.37125492237,126.72207822482,7.9044,22.3000,-0.0192,0.2821,0.0128,-1.302544684,0.456729396,88.350488881,0.4069,0.2763,0.5124,0.1098,0.0900,0.0754,0.1799,0.1848,5.1698,0f000001,0*d36670cb\n\tsystem status\tnormal 2 28.200000 0 0\trobot status\t110.113509\t124.826528\t7.904400\t-1.302545\t0.456729\t1.649511\t0.335000\t-0.063000\n\t\n15:12:02.4\tlog_raw\tgps_raw\t#INSPVAXA,USB3,0,49.0,FINESTEERING,2107,281540.450,02000000,471d,15824;INS_ALIGNMENT_COMPLETE,INS_RTKFIXED,37.37125492050,126.72207986895,7.9075,22.3000,-0.0253,0.2731,0.0097,-1.293452361,0.411042124,88.411048342,0.4069,0.2763,0.5116,0.1099,0.0902,0.0754,0.1799,0.1848,5.1684,0f000001,0*2b0ddc64\n\tsystem status\tnormal 2 28.200000 0 0\trobot status\t110.259144\t124.826318\t7.907500\t-1.293452\t0.411042\t1.588952\t0.286000\t0.005000\n\t\n15:12:02.9\tlog_raw\tgps_raw\t\tsystem status\tnormal 2 28.200000 0 0\trobot status\t110.401167\t124.824667\t7.911500\t-1.158295\t0.398518\t1.581312\t0.303000\t0.000000\n\t\n15:12:03.4\tlog_raw\tgps_raw\t\tsystem status\tnormal 2 28.200000 0 0\trobot status\t110.541862\t124.823109\t7.915000\t-1.102689\t0.293589\t1.544269\t0.295000\t-0.002000\n\t\n15:12:03.9\tlog_raw\tgps_raw\t#INSPVAXA,USB3,0,48.5,FINESTEERING,2107,281541.950,02000000,471d,15824;INS_ALIGNMENT_COMPLETE,INS_RTKFIXED,37.37125486975,126.72208463852,7.9183,22.3000,-0.0254,0.2525,0.0080,-1.001794555,0.208047593,88.595435121,0.4068,0.2761,0.5109,0.1098,0.0900,0.0754,0.1799,0.1848,5.1663,0f000001,0*dcb79567\n\tsystem status\tnormal 2 28.200000 0 0\trobot status\t110.681624\t124.820680\t7.918300\t-1.001795\t0.208048\t1.404565\t0.291000\t-0.050000\n\t\n15:12:04.4\tlog_raw\tgps_raw\t#INSPVAXA,USB3,0,49.0,FINESTEERING,2107,281542.450,02000000,471d,15824;INS_ALIGNMENT_COMPLETE,INS_RTKFIXED,37.37125484773,126.72208610696,7.9206,22.3000,-0.0083,0.3427,0.0268,-0.912942470,0.207155867,88.931332893,0.4067,0.2761,0.5105,0.1096,0.0899,0.0754,0.1798,0.1848,5.1642,0f000001,0*e5dcf027\n\tsystem status\tnormal 2 28.200000 0 0\trobot status\t110.811696\t124.818235\t7.920600\t-0.912942\t0.207156\t1.068667\t0.296000\t-0.080000\n\t\n15:12:04.9\tlog_raw\tgps_raw\t\tsystem status\tnormal 2 28.200000 0 0\trobot status\t110.977481\t124.816579\t7.923000\t-0.893782\t0.039069\t1.037062\t0.281000\t0.195000\n\t\n15:12:05.4\tlog_raw\tgps_raw\t\tsystem status\tnormal 2 27.800000 0 0\trobot status\t111.117192\t124.815027\t7.926800\t-0.631344\t0.046007\t2.815440\t0.271000\t0.137000\n\t\n15:12:05.9\tlog_raw\tgps_raw\t#INSPVAXA,USB3,0,49.5,FINESTEERING,2107,281543.950,02000000,471d,15824;INS_ALIGNMENT_COMPLETE,INS_RTKFIXED,37.37125492276,126.72209111825,7.9296,22.3000,0.0316,0.2804,0.0153,-0.692370784,0.020659336,82.875038153,0.4068,0.2761,0.5102,0.1095,0.0899,0.0754,0.1798,0.1847,5.1628,0f000001,0*67f5d293\n\tsystem status\tnormal 2 27.300000 0 0\trobot status\t111.255588\t124.826556\t7.929600\t-0.692371\t0.020659\t7.124962\t0.275000\t0.208000\n\t\n15:12:06.4\tlog_raw\tgps_raw\t#INSPVAXA,USB3,0,50.0,FINESTEERING,2107,281544.450,02000000,471d,15824;INS_ALIGNMENT_COMPLETE,INS_RTKFIXED,37.37125505566,126.72209271509,7.9316,22.3000,0.0505,0.2738,0.0268,-0.616767786,0.154143258,78.067707223,0.4067,0.2763,0.5098,0.1099,0.0900,0.0754,0.1797,0.1847,5.1619,0f000001,0*4337cbac\n\tsystem status\tnormal 2 27.500000 4 0\trobot status\t111.397034\t124.841304\t7.931600\t-0.616768\t0.154143\t11.932293\t0.265000\t0.178000\n\t\n15:12:06.9\tlog_raw\tgps_raw\t\tsystem status\tnormal 2 27.400000 4 0\trobot status\t111.537278\t124.870947\t7.932800\t-0.497230\t0.092847\t16.005246\t0.294000\t0.126000\n\t\n15:12:07.4\tlog_raw\tgps_raw\t#INSPVAXA,USB3,0,47.5,FINESTEERING,2107,281545.450,02000000,471d,15824;INS_ALIGNMENT_COMPLETE,INS_RTKFIXED,37.37125567911,126.72209586319,7.9361,22.3000,0.0734,0.2704,0.0174,-0.731540413,0.133149102,70.486374677,0.4064,0.2767,0.5097,0.1103,0.0911,0.0753,0.1798,0.1847,5.1599,0f000001,0*4759ac49\n\tsystem status\tnormal 2 27.500000 4 0\trobot status\t111.675887\t124.910493\t7.936100\t-0.731540\t0.133149\t19.513625\t0.303000\t0.117000\n\t\n15:12:07.9\tlog_raw\tgps_raw\t#INSPVAXA,USB3,0,47.5,FINESTEERING,2107,281545.950,02000000,471d,15824;INS_ALIGNMENT_COMPLETE,INS_RTKFIXED,37.37125607129,126.72209738757,7.9408,22.3000,0.0944,0.2605,0.0183,-0.696019275,0.088406772,68.352521751,0.4064,0.2767,0.5097,0.1103,0.0911,0.0753,0.1798,0.1847,5.1599,0f000001,0*d303d9f5\n\tsystem status\tnormal 2 27.600000 4 0\trobot status\t111.810914\t124.954018\t7.940800\t-0.696019\t0.088407\t21.647478\t0.301000\t0.076000\n\t\n15:12:08.4\tlog_raw\tgps_raw\t#INSPVAXA,USB3,0,49.0,FINESTEERING,2107,281546.450,02000000,471d,15824;INS_ALIGNMENT_COMPLETE,INS_RTKFIXED,37.37125652974,126.72209892700,7.9445,22.3000,0.1147,0.2632,0.0224,-0.803440869,0.020202834,66.760557028,0.4064,0.2770,0.5100,0.1115,0.0928,0.0753,0.1798,0.1846,5.1557,0f000001,0*6d000163\n\tsystem status\tnormal 2 27.600000 4 0\trobot status\t111.947274\t125.004897\t7.944500\t-0.803441\t0.020203\t23.239443\t0.310000\t0.029000\n\t\n15:12:08.9\tlog_raw\tgps_raw\t\tsystem status\tnormal 2 27.800000 0 0\trobot status\t112.082192\t125.059018\t7.946200\t-0.982611\t0.080093\t24.189594\t0.310000\t0.006000\n\t\n15:12:09.4\tlog_raw\tgps_raw\t\tsystem status\tnormal 2 28.100000 0 0\trobot status\t112.218345\t125.113233\t7.944300\t-1.137554\t0.128945\t24.460920\t0.395000\t-0.147000\n\t\n15:12:09.9\tlog_raw\tgps_raw\t#INSPVAXA,USB3,0,51.5,FINESTEERING,2107,281547.950,02000000,471d,15824;INS_ALIGNMENT_COMPLETE,INS_RTKFIXED,37.37125797695,126.72210352475,7.9421,22.3000,0.1103,0.2645,0.0073,-1.143829533,0.094704547,65.656045982,0.4068,0.2775,0.5101,0.1136,0.0952,0.0753,0.1797,0.1843,5.1506,0f000001,0*3e76ed6a\n\tsystem status\tnormal 2 28.200000 0 0\trobot status\t112.354536\t125.165509\t7.942100\t-1.143830\t0.094705\t24.343954\t0.341000\t-0.079000\n\t\n15:12:10.4\tlog_raw\tgps_raw\t#INSPVAXA,USB3,0,46.5,FINESTEERING,2107,281548.450,02000000,471d,15824;INS_ALIGNMENT_COMPLETE,INS_RTKFIXED,37.37125842194,126.72210499734,7.9414,22.3000,0.0987,0.2565,0.0113,-1.211419516,0.114110023,65.814844612,0.4000,0.2752,0.5002,0.1145,0.0964,0.0745,0.1794,0.1832,5.1447,0f000001,0*e7619ae9\n\tsystem status\tnormal 2 28.200000 0 0\trobot status\t112.484975\t125.214895\t7.941400\t-1.211420\t0.114110\t24.185155\t0.302000\t-0.062000\n\t\n15:12:10.9\tlog_raw\tgps_raw\t\tsystem status\tnormal 2 28.200000 0 0\trobot status\t112.611166\t125.260300\t7.940800\t-1.226777\t0.195265\t23.882750\t0.298000\t-0.059000\n\t\n15:12:11.4\tlog_raw\tgps_raw\t\tsystem status\tnormal 2 28.100000 0 0\trobot status\t112.766577\t125.318747\t7.939900\t-1.431004\t-0.036678\t23.280479\t0.302000\t-0.039000\n\t\n15:12:11.9\tlog_raw\tgps_raw\t\tsystem status\tnormal 2 28.000000 0 0\trobot status\t112.908210\t125.365462\t7.939500\t-1.309759\t-0.246709\t21.917425\t0.371000\t0.031000\n\t\n15:12:12.4\tlog_raw\tgps_raw\t#INSPVAXA,USB3,0,50.0,FINESTEERING,2107,281550.450,02000000,471d,15824;INS_ALIGNMENT_COMPLETE,INS_RTKFIXED,37.37126014909,126.72211137085,7.9382,22.3000,0.0775,0.2990,0.0098,-1.324688179,-0.327901204,70.475818892,0.4093,0.2808,0.5055,0.1189,0.0988,0.0751,0.1779,0.1804,5.1364,0f000001,0*808235da\n\tsystem status\tnormal 2 27.600000 0 0\trobot status\t113.049530\t125.406574\t7.938200\t-1.324688\t-0.327901\t19.524181\t0.291000\t-0.106000\n\t\n15:12:12.9\tlog_raw\tgps_raw\t#INSPVAXA,USB3,0,50.0,FINESTEERING,2107,281550.950,02000000,471d,15824;INS_ALIGNMENT_COMPLETE,INS_RTKFIXED,37.37126045851,126.72211301062,7.9366,22.3000,0.0692,0.2949,0.0149,-1.528450256,-0.256130387,73.623851068,0.4093,0.2808,0.5055,0.1189,0.0988,0.0751,0.1779,0.1804,5.1364,0f000001,0*9b441f42\n\tsystem status\tnormal 2 27.600000 0 0\trobot status\t113.194778\t125.440913\t7.936600\t-1.528450\t-0.256130\t16.376149\t0.300000\t-0.131000\n\t\n15:12:13.4\tlog_raw\tgps_raw\t#INSPVAXA,USB3,0,50.5,FINESTEERING,2107,281551.450,02000000,471d,15824;INS_ALIGNMENT_COMPLETE,INS_RTKFIXED,37.37126071585,126.72211464730,7.9349,22.3000,0.0461,0.2986,0.0130,-1.521992533,-0.266379838,76.609836903,0.4123,0.2823,0.5064,0.1185,0.0974,0.0752,0.1766,0.1780,5.1359,0f000001,0*10c7b170\n\tsystem status\tnormal 2 27.500000 0 0\trobot status\t113.339753\t125.469472\t7.934900\t-1.521993\t-0.266380\t13.390163\t0.297000\t-0.126000\n\t\n15:12:13.9\tlog_raw\tgps_raw\t\tsystem status\tnormal 2 27.400000 0 0\trobot status\t113.485707\t125.490275\t7.933600\t-1.562849\t0.127250\t10.517474\t0.281000\t-0.087000\n\t\n15:12:14.4\tlog_raw\tgps_raw\t\tsystem status\tnormal 2 27.500000 4 0\trobot status\t113.631100\t125.499963\t7.932600\t-1.190061\t0.385237\t7.912451\t0.310000\t-0.082000\n\t\n15:12:14.9\tlog_raw\tgps_raw\t\tsystem status\tnormal 2 27.700000 4 0\trobot status\t113.777886\t125.503423\t7.931900\t-0.973669\t0.545202\t5.593259\t0.289000\t-0.069000\n\t\n15:12:15.4\tlog_raw\tgps_raw\t#INSPVAXA,USB3,0,46.0,FINESTEERING,2107,281553.450,02000000,471d,15824;INS_ALIGNMENT_COMPLETE,INS_RTKFIXED,37.37126103128,126.72212124839,7.9298,22.3000,-0.0140,0.3127,0.0103,-1.123324065,0.508186608,86.475443339,0.4150,0.2827,0.5081,0.1139,0.0931,0.0752,0.1739,0.1735,5.1368,0f000001,0*51a33212\n\tsystem status\tnormal 2 27.700000 4 0\trobot status\t113.924467\t125.504472\t7.929800\t-1.123324\t0.508187\t3.524557\t0.296000\t-0.059000\n\t\n15:12:15.9\tlog_raw\tgps_raw\t#INSPVAXA,USB3,0,46.0,FINESTEERING,2107,281553.950,02000000,471d,15824;INS_ALIGNMENT_COMPLETE,INS_RTKFIXED,37.37126097435,126.72212290595,7.9280,22.3000,-0.0108,0.3087,0.0193,-0.994058231,0.235221833,88.104277640,0.4150,0.2827,0.5081,0.1139,0.0931,0.0752,0.1739,0.1735,5.1368,0f000001,0*a2074ee6\n\tsystem status\tnormal 2 27.900000 0 0\trobot status\t114.071291\t125.498151\t7.928000\t-0.994058\t0.235222\t1.895722\t0.303000\t-0.043000\n\t\n15:12:16.4\tlog_raw\tgps_raw\t\tsystem status\tnormal 2 27.900000 0 0\trobot 
